vi "CheckLastConnect.vi"(8 "error in (no error)":errorcluster, 11 "GiaoTiepUART in":refnum<class "GiaoTiepUART.lvclass">) -> (0 "error out":errorcluster, 2 "timeOut":bool, 3 "GiaoTiepUART out":refnum<class "GiaoTiepUART.lvclass">)   [LabVIEW 2017, in "LibraryGcode.lvlib" / "GiaoTiepUART.lvclass"]
uses:
  GiaoTiepUART.lvclass
  GiaoTiepUART.lvclass/GiaoTiepUART.ctl
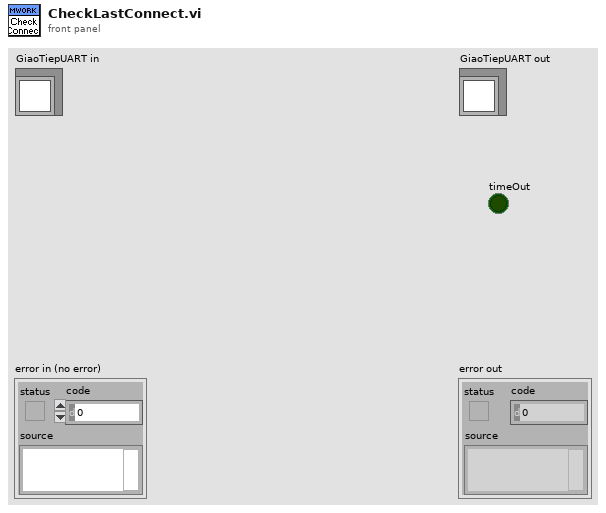
[diagram p1: front panel]
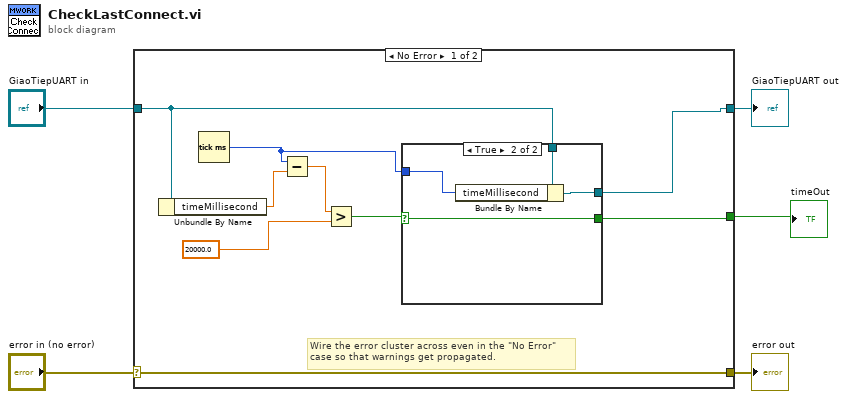
[diagram p0: block diagram]
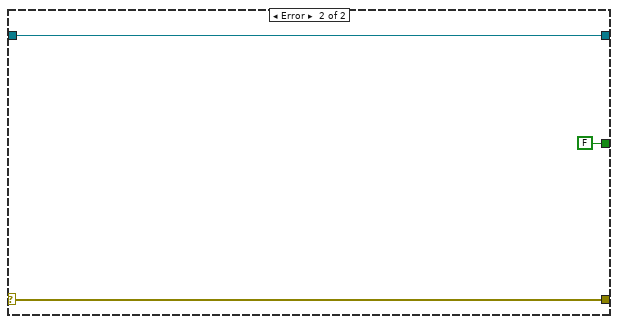
[diagram p3: hidden frame]
diagram:
  n1 = case shown="No Error" "error in (no error)" {
    selector: "error in (no error)" -> [w14 w23]
    tunnel: [w14 w23] -> w4
    tunnel: [w7 w22] -> w2
    tunnel: "GiaoTiepUART in" -> [w8 w22]
    tunnel: [w9 FALSE] -> w1
    frame No Error {
      # "Wire the error cluster across even in the \"No Error\"\ncase so that warnings get propagated."
      n2 = Unbundle By Name(w8) -> ("timeMillisecond"=w13:dbl)
      n3 = Tick Count (ms)() -> (millisecond timer value=w6:u32)
      n4 = Subtract(x=w6, y=w13) -> (x-y=w12:dbl)
      n5 = Greater?(x=w12, y=20000.0) -> (0:w10:bool)
      n6 = case shown="True" w10 {
        selector: w10 -> [w16 w20]
        tunnel: [w16 w20] -> w9
        tunnel: w8 -> [w15 w19]
        tunnel: [w15 w18] -> w7
        tunnel: w6 -> [_ w17]
        frame False {
        }
        frame True {
          n7 = Bundle By Name(cluster=w19, "timeMillisecond"=w17) -> (w18:refnum<class "GiaoTiepUART.lvclass">)
        }
      }
    }
    frame Error {
    }
  }
  "error out" <- w4
  "GiaoTiepUART out" <- w2
  "timeOut" <- w1
